vi "MAX5217 Write.vi"(6 "error in (no error)":errorcluster, 8 "DAC code":u16, 9 "VISA Refnum in":refnum<visa-resource-name>) -> (0 "error out":errorcluster, 3 "VISA Refnum out":refnum<visa-resource-name>)   [LabVIEW 2015]
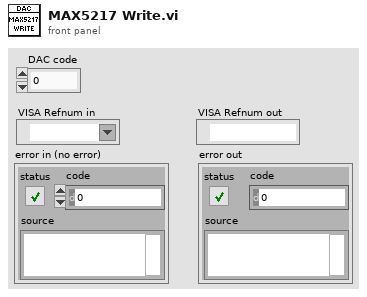
[diagram p1: front panel]
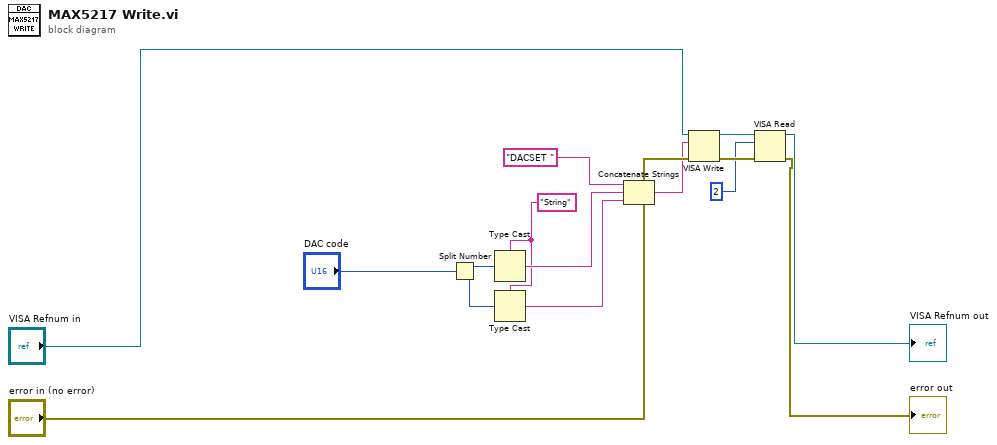
[diagram p0: block diagram]
diagram:
  w2 = "String" ("type")
  n1 = Split Number(x="DAC code") -> (hi(x)=w7:u8, lo(x)=w5:u8)
  n2 = Type Cast(type=w2, x=w7) -> (*(type *) &x=w3:string)
  n3 = Type Cast(type=w2, x=w5) -> (*(type *) &x=w6:string)
  n4 = Concatenate Strings("DACSET " ("string"), w3, w6) -> (w12:string)
  n5 = VISA Write(VISA resource name="VISA Refnum in", write buffer=w12, error in (no error)="error in (no error)") -> (VISA resource name out=w11:refnum<visa-resource-name>, error out=w10:errorcluster)  [unwired: 1 out]
  n6 = VISA Read(VISA resource name=w11, byte count=u32 2, error in (no error)=w10) -> (VISA resource name out=→"VISA Refnum out":refnum<visa-resource-name>, error out=→"error out":errorcluster)  [unwired: 2 out]
